vi "Main.vi"() -> ()   [LabVIEW 2016]
uses:
  <vilib>/Utility/error.llb/DialogType.ctl
  <vilib>/Utility/file.llb/Write Delimited Spreadsheet (string).vi
  <vilib>/Analysis/2dsp.llb/Rational Resample (single channel, DBL).vi
  <vilib>/measure/mamon.llb/Trigger Detection for 1 Channel.vi
  <vilib>/measure/NI_MAPro.lvlib
  <vilib>/Analysis/NI_AALPro.lvlib
panel:
  out "Waveform Graph":dbl[](graph)
  out "Y":dbl[](array[numeric])
  out "Software Version":string
  in  "Tab Control 2":enum32{"Calculated Values", "Other Values"}(tab)
  out "Contraction\nOnset (s)":dbl format="%_5g"
  out "Standing\nWeight":dbl format="%.1f"
  out "Peak Force":dbl format="%.1f"
  out "Mean Force":dbl format="%.1f"
  out "Min Force":dbl format="%.1f"
  out "TTPF":dbl format="%_5g"
  out "RFDPF":dbl format="%.1f"
  out "IMPPF":dbl format="%.1f"
  out "IMP250":dbl format="%_5g"
  out "IMP200":dbl format="%_5g"
  out "IMP150":dbl format="%_5g"
  out "IMP100":dbl format="%_5g"
  out "RFD250":dbl format="%.1f"
  out "RFD200":dbl format="%.1f"
  out "RFD150":dbl format="%.1f"
  out "RFD100":dbl format="%.1f"
  out "F250":dbl format="%.1f"
  out "F200":dbl format="%.1f"
  out "F150":dbl format="%.1f"
  out "F100":dbl format="%.1f"
  out "System Weight \nCursor Position":dbl
  out "Before Pull Cursor\nPosition":dbl
  out "After pull\nCursor Position":dbl
  out "SD of weighing period":dbl format="%#_4g"
  in  "stop 2":bool
  out "Index of min SD":dbl format="%#.2f"
  out "Minimum SD":dbl
  in  "Tab Control 3":T1(tab)
  out "Peak Deviation >50N\nfrom Average?":bool
  out "System Weight Segment":dynamicdata(graph)
  out "SW Segment Range":dbl
  out "Contraction Onset ID":dbl[](graph) caption="Section"
  out "Intra-Cursor Segment":dbl[](graph)
  in  "Tab Control":T2(tab)
  in  "Subject Body Mass (kg)":dbl
  in  "Subject Identifier (ID# or Last Name, First)":string
  in  "Trial Number":string
  in  "Trial Notes":string
  in  "Create Blank\nSave File":bool
  in  "Save Results":bool
  out "Target File for Saving Results":path
  in  "Choose New \nSave Target":bool
  out "Analysis File and File Path":path
  in  "Load File":bool
  in  "Sampling Rate\nof Force Signal":i32=100 min=100 max=2000 step=1 format="%#.0f"
  in  "Custom Onset Threshold\nValue in Newtons (SW+Threshold)":dbl min=0.0 max=500.0
  in  "# of Samples Averaged for system \nweight (Default is 1000).":i32=1000 caption="Samples" min=3 max=2000
  in  "Suppress \nData Prompt":bool
  in  "Contraction Onset ID Method":u16(ring) items=["5SD of Weighing", "20 N", "75 N", "Manual Identification", "Custom Threshold"]
  out "Force-time trace":dynamicdata(graph)
  # "Isometric Analyzer\nBy George Beckham, PhD"
  # "Main Github Repository: \nhttps://github.com/excellentsport/IsometricAnalyzer"
  # "This is beta version software, and may have bugs. \nPlease submit any that you find at: \nhttps://github.com/excellentsport/IsometricAnalyzer/issues"
  # "How to use: \nhttps://github.com/excellentsport/IsometricAnalyzer"
  # "All values displayed above are assumed to operate using Newtons as the unit of force. Hence, all boxes with force are\nin Newtons, all Rate of Force Development (RFD) are in Newtons per second (N/s), and Impulse (IMP) is in N•s.\n\nEach time specific value (e.g. F100) is calculated relative to the contraction onset (e.g. F100 is the force at 100ms after the contraction began)."
  # "Horizontal line is SW value"
  # "Green Cursor Designates the identified start of the push/pull\nRed Cursor Designates the identified end of the push/pull"
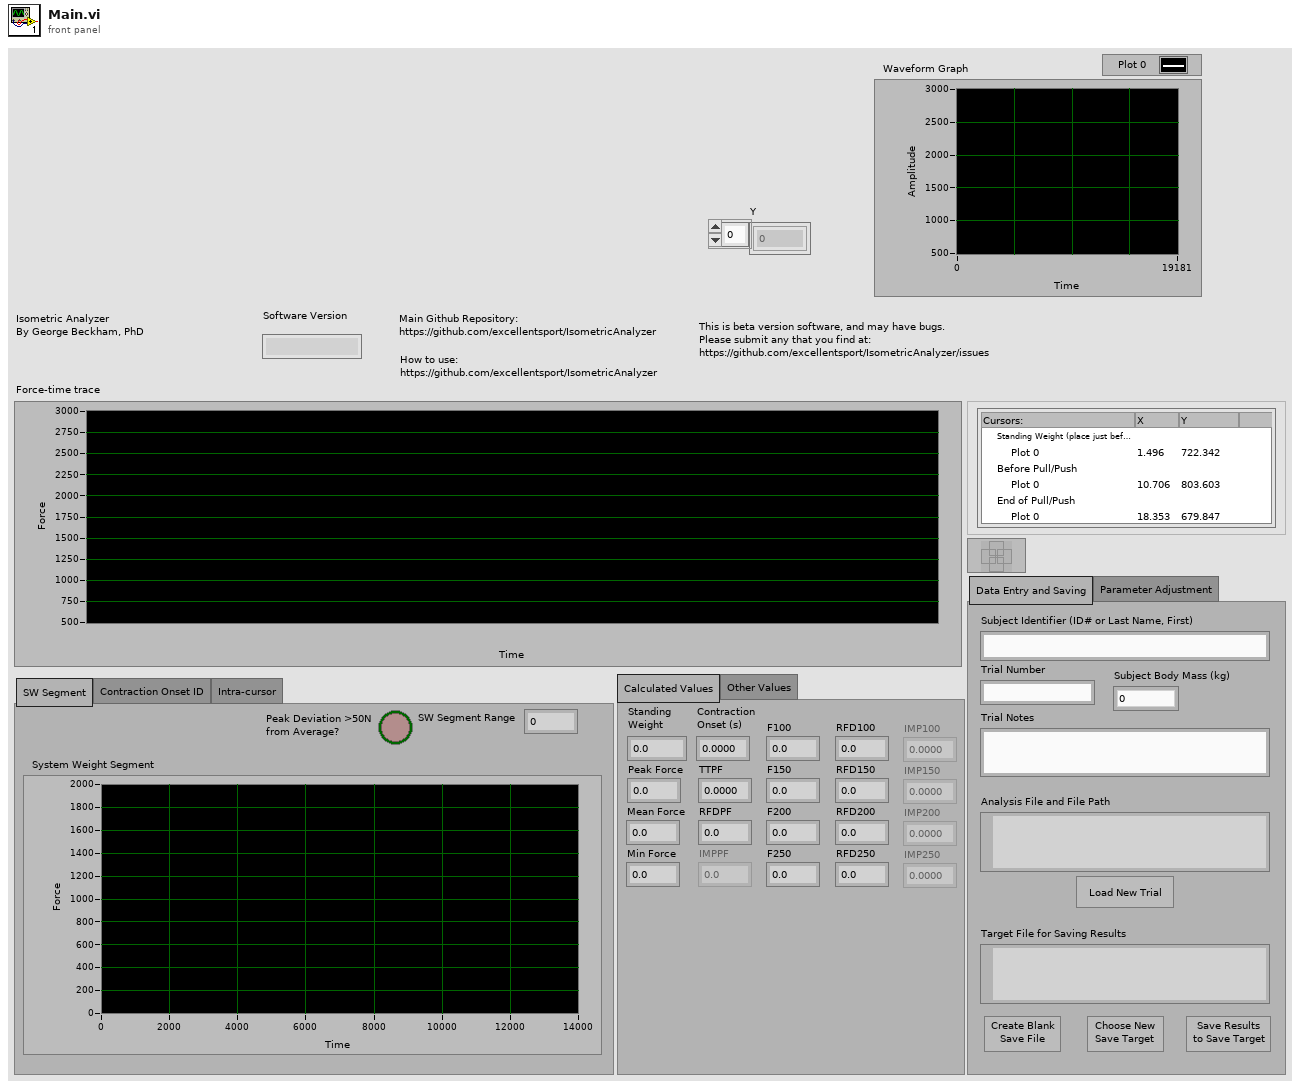
[diagram p1: front panel]
types:
  T1 = enum32{"SW Segment", "Contraction Onset ID", "Intra-cursor"}
  T2 = enum32{"Data Entry and Saving", "Parameter Adjustment"}
  T3 = typedef "DialogType.ctl" = u16
  T4 = cluster{i32, "Sampling Rate\nof Force Signal":i32}
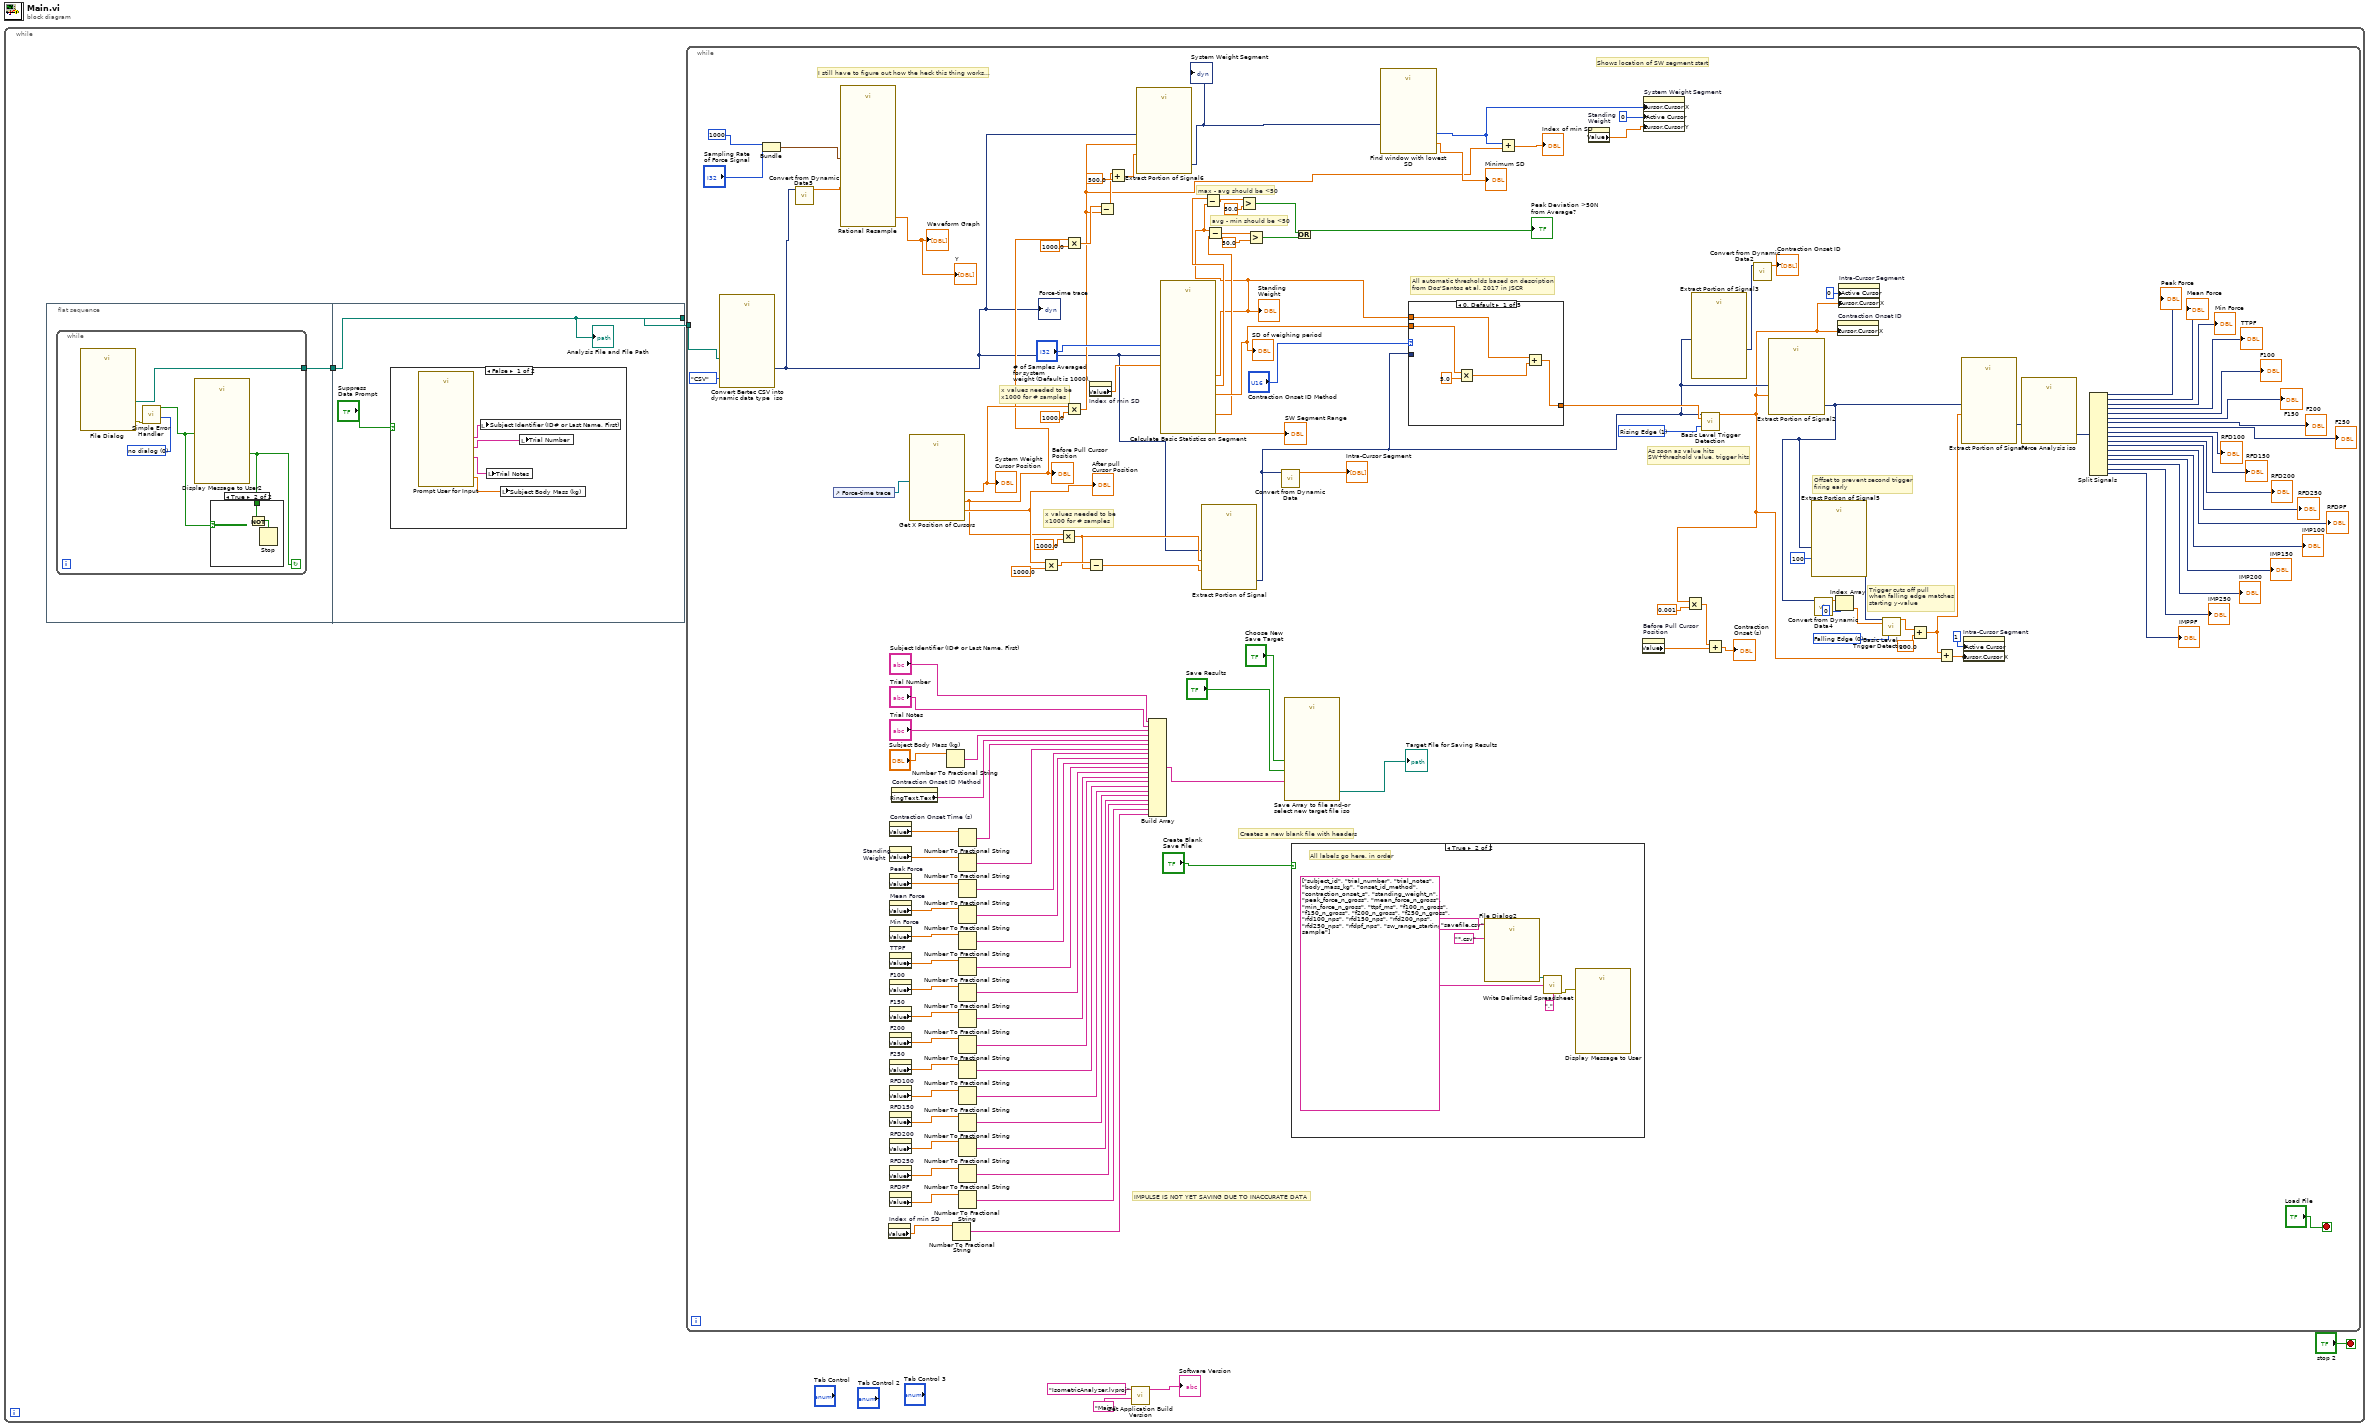
[diagram p0: block diagram]
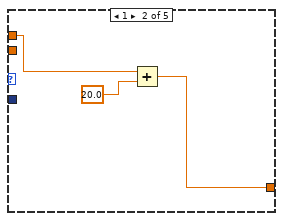
[diagram p4: hidden frame]
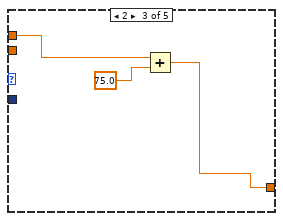
[diagram p5: hidden frame]
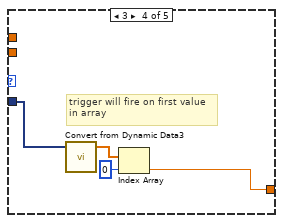
[diagram p6: hidden frame]
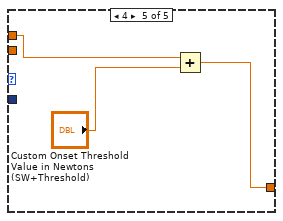
[diagram p7: hidden frame]
diagram:
  n1 = while {
    stop <- "stop 2" stop-if-true
    n2 = flat-sequence {
      tunnel: [w7] -> w1
      tunnel: [w15] -> w6
      tunnel: w1 -> [w15]
      frame #0 {
        n3 = while {
          tunnel: [w12] -> w7
          stop <- w9 continue-if-true
          w10 = T3 0 items=["no dialog", "OK message", "continue or stop message", "OK message + warnings", "continue/stop + warnings"] ("type of dialog (OK msg:1)")
          n4 = call "File Dialog"() -> ("selected path"=w12:path, "error out"=w11:errorcluster)  [unwired: 12 in, 2 out]
          n5 = call <vilib>:"Simple Error Handler.vi"("type of dialog (OK msg:1)"=w10, "error in (no error)"=w11) -> ("error?"=w8:bool)  [unwired: 3 in, 4 out]
          n6 = call "Display Message to User2"("Enable"=w8) -> ("OK"=w9:bool)  [unwired: 9 in, 1 out]
          n7 = case shown="True" w8 {
            tunnel: w9 -> [_ w13]
            frame False {
            }
            frame True {
              n8 = Not(x=w13) -> (.not. x?=w14:bool)
              n9 = Stop(stop? (T)=w14) -> ()
            }
          }
        }
      }
      frame #1 {
        n10 = case shown="False" "Suppress \nData Prompt" {
          frame False {
            n11 = call "Prompt User for Input"() -> ("Subject's body mass (kg)"=w17:dbl, "Trial Notes"=w19:string, "Trial Number"=w18:string, "Subject ID (e.g. 007) or Last Name, First Name"=w20:string)  [unwired: 14 in, 2 out]
            n12 = local write "Subject Identifier (ID# or Last Name, First)"(w20) -> ()
            n13 = local write "Trial Notes"(w19) -> ()
            n14 = local write "Subject Body Mass (kg)"(w17) -> ()
            n15 = local write "Trial Number"(w18) -> ()
          }
          frame True {
          }
        }
        "Analysis File and File Path" <- w15
      }
    }
    n16 = while {
      tunnel: w6 -> [w152]
      stop <- "Load File" stop-if-true
      w86 = u16 0 items=["Falling Edge", "Rising Edge"] ("trigger slope")
      w89 = u16 1 items=["Falling Edge", "Rising Edge"] ("trigger slope")
      # "I still have to figure out how the heck this thing works..."
      # "Shows location of SW segment start"
      # "Offset to prevent second trigger\nfiring early"
      # "avg - min should be <50"
      # "max - avg should be <50"
      # "All automatic thresholds based on description \nfrom Dos'Santos et al. 2017 in JSCR"
      # "Trigger cuts off pull\nwhen falling edge matches \nstarting y-value"
      # "As soon as value hits \nSW+threshold value, trigger hits"
      # "IMPULSE IS NOT YET SAVING DUE TO INACCURATE DATA"
      # "Creates a new blank file with headers"
      # "x values needed to be \nx1000 for # samples"
      # "x values needed to be \nx1000 for # samples"
      n17 = call "Convert Bertec CSV into dynamic data type  iso.vi"("selected path"=w152, "Input Datafile Separator"=enum32{"CSV", "TSV"}."CSV" ("Input Datafile Type")) -> ("Dynamic Data Type"=w26:dynamicdata)
      "Force-time trace" <- w26
      n18 = Bundle(1000, "Sampling Rate\nof Force Signal"="Sampling Rate\nof Force Signal") -> (w22:T4)  [unwired: 1 in]
      n19 = call "Convert from Dynamic Data5"("Dynamic Data Type"=w26) -> ("Array"=w25:dbl[])  [unwired: 3 in]
      n20 = control-ref of="Force-time trace"() -> (w150:refnum<vi>)
      n21 = call-poly <vilib>:"Rational Resample.vi"("resample factor"=w22, "X"=w25) -> ("Y"=→"Y" →"Waveform Graph":dbl[])  [unwired: 7 in, 2 out]
      n22 = property on="Index of min SD" class="DigNum (strict)"() -> ("Value"=w28:dbl)  [unwired: 2 in, 2 out]
      n23 = property on="Contraction Onset Time (s)" class="DigNum (strict)"() -> ("Value"=w61:dbl)  [unwired: 2 in, 2 out]
      n24 = property on="Standing\nWeight" class="DigNum (strict)"() -> ("Value"=w94:dbl)  [unwired: 2 in, 2 out]
      n25 = property on="Peak Force" class="DigNum (strict)"() -> ("Value"=w120:dbl)  [unwired: 2 in, 2 out]
      n26 = property on="Mean Force" class="DigNum (strict)"() -> ("Value"=w118:dbl)  [unwired: 2 in, 2 out]
      n27 = property on="Min Force" class="DigNum (strict)"() -> ("Value"=w117:dbl)  [unwired: 2 in, 2 out]
      n28 = property on="TTPF" class="DigNum (strict)"() -> ("Value"=w116:dbl)  [unwired: 2 in, 2 out]
      n29 = property on="F100" class="DigNum (strict)"() -> ("Value"=w115:dbl)  [unwired: 2 in, 2 out]
      n30 = property on="F150" class="DigNum (strict)"() -> ("Value"=w114:dbl)  [unwired: 2 in, 2 out]
      n31 = property on="F200" class="DigNum (strict)"() -> ("Value"=w113:dbl)  [unwired: 2 in, 2 out]
      n32 = property on="F250" class="DigNum (strict)"() -> ("Value"=w112:dbl)  [unwired: 2 in, 2 out]
      n33 = property on="RFD100" class="DigNum (strict)"() -> ("Value"=w111:dbl)  [unwired: 2 in, 2 out]
      n34 = property on="RFD150" class="DigNum (strict)"() -> ("Value"=w110:dbl)  [unwired: 2 in, 2 out]
      n35 = property on="RFD200" class="DigNum (strict)"() -> ("Value"=w109:dbl)  [unwired: 2 in, 2 out]
      n36 = property on="RFD250" class="DigNum (strict)"() -> ("Value"=w108:dbl)  [unwired: 2 in, 2 out]
      n37 = property on="RFDPF" class="DigNum (strict)"() -> ("Value"=w107:dbl)  [unwired: 2 in, 2 out]
      n38 = property on="Contraction Onset ID Method" class="Ring (strict)"() -> ("RingText.Text"=w52:string)  [unwired: 2 in, 2 out]
      n39 = call "Get X Position of Cursors.vi"("WaveformGraph in"=w150) -> ("Cursor 3 X Pos"=w91:dbl, "Cursor 2 X Pos"=w40:dbl, "Cursor 1 X Pos"=w92:dbl)  [unwired: 7 in]
      "After pull\nCursor Position" <- w91
      "Before Pull Cursor\nPosition" <- w40
      "System Weight \nCursor Position" <- w92
      n40 = Number To Fractional String(number="Subject Body Mass (kg)") -> (F-format string=w54:string)  [unwired: 3 in]
      n41 = Number To Fractional String(number=w28) -> (F-format string=w27:string)  [unwired: 3 in]
      n42 = Number To Fractional String(number=w61) -> (F-format string=w60:string)  [unwired: 3 in]
      n43 = Number To Fractional String(number=w94) -> (F-format string=w82:string)  [unwired: 3 in]
      n44 = Number To Fractional String(number=w120) -> (F-format string=w119:string)  [unwired: 3 in]
      n45 = Number To Fractional String(number=w118) -> (F-format string=w106:string)  [unwired: 3 in]
      n46 = Number To Fractional String(number=w117) -> (F-format string=w105:string)  [unwired: 3 in]
      n47 = Number To Fractional String(number=w116) -> (F-format string=w104:string)  [unwired: 3 in]
      n48 = Number To Fractional String(number=w115) -> (F-format string=w103:string)  [unwired: 3 in]
      n49 = Number To Fractional String(number=w114) -> (F-format string=w102:string)  [unwired: 3 in]
      n50 = Number To Fractional String(number=w113) -> (F-format string=w101:string)  [unwired: 3 in]
      n51 = Number To Fractional String(number=w112) -> (F-format string=w100:string)  [unwired: 3 in]
      n52 = Number To Fractional String(number=w111) -> (F-format string=w99:string)  [unwired: 3 in]
      n53 = Number To Fractional String(number=w110) -> (F-format string=w98:string)  [unwired: 3 in]
      n54 = Number To Fractional String(number=w109) -> (F-format string=w97:string)  [unwired: 3 in]
      n55 = Number To Fractional String(number=w108) -> (F-format string=w96:string)  [unwired: 3 in]
      n56 = Number To Fractional String(number=w107) -> (F-format string=w95:string)  [unwired: 3 in]
      n57 = Multiply(x=w91, y=1000.0) -> (x*y=w146:dbl)
      n58 = Multiply(x=w40, y=1000.0) -> (x*y=w42:dbl)
      n59 = Multiply(x=w40, y=1000.0) -> (x*y=w38:dbl)
      n60 = Multiply(x=w92, y=1000.0) -> (x*y=w36:dbl)
      n61 = Subtract(x=w146, y=w42) -> (x-y=w145:dbl)
      n62 = property on="Index of min SD" class="DigNum (strict)"() -> ("Value"=w34:dbl)  [unwired: 2 in, 2 out]
      n63 = Subtract(x=w38, y=w36) -> (x-y=w41:dbl)
      n64 = Add(x=w41, y=500.0) -> (x+y=w44:dbl)
      n65 = call "Extract Portion of Signal6"("Samples"=w44, "Begin Sample"=w36, "Signals"=w26) -> ("Section"=w33:dynamicdata)  [unwired: 7 in, 1 out]
      "System Weight Segment" <- w33
      n66 = Build Array("Subject Identifier (ID# or Last Name, First)", "Trial Number", "Trial Notes", w54, w52, w60, w82, w119, w106, w105, w104, w103, w102, w101, w100, w99, w98, w97, w96, w95, w27) -> (w123:string[])
      n67 = call "Calculate Basic Statistics on Segment.vi"("# of Samples Averaged\nfor standing weight\n(1000 is default)"="# of Samples Averaged for system \nweight (Default is 1000).", "Start of Sample"=w34, "Dynamic Data Type"=w26) -> ("Minimum"=w70:dbl, "Maximum"=w69:dbl, "Standard Deviation"=w83:dbl, "Arithmetic Mean"=w29:dbl, "Range"=→"SW Segment Range":dbl)  [unwired: 3 in, 1 out]
      "Standing\nWeight" <- w29
      "SD of weighing period" <- w83
      n68 = call "Extract Portion of Signal"("Samples"=w145, "Begin Sample"=w42, "Signals"=w26) -> ("Section"=w79:dynamicdata)  [unwired: 7 in, 1 out]
      n69 = Subtract(x=w69, y=w29) -> (x-y=w71:dbl)
      n70 = Subtract(x=w29, y=w70) -> (x-y=w66:dbl)
      n71 = Greater?(x=w71, y=50.0) -> (0:w73:bool)
      n72 = Greater?(x=w66, y=50.0) -> (0:w68:bool)
      n73 = call "Convert from Dynamic Data"("Dynamic Data Type"=w79) -> ("Array"=→"Intra-Cursor Segment":dbl[])  [unwired: 3 in]
      n74 = call "Save Array to file and-or select new target file iso.vi"("Choose New \nSave Target"="Choose New \nSave Target", "Save Results"="Save Results", "Values to Save"=w123) -> ("selected path"=→"Target File for Saving Results":path)  [unwired: 8 in]
      n75 = case shown="True" "Create Blank\nSave File" {
        frame False {
        }
        frame True {
          # "All labels go here, in order"
          n76 = call "File Dialog2"("default name"="savefile.csv", "pattern (all files)"="*.csv") -> ("selected path"=w174:path)  [unwired: 10 in, 3 out]
          n77 = call-poly <vilib>:"Write Delimited Spreadsheet.vi"("file path (dialog if empty)"=w174, "1D data"=string[] ["subject_id", "trial_number", "trial_notes", "body_mass_kg", "onset_id_method", "contraction_onset_s", "standing_weight_n", "peak_force_n_gross", "mean_force_n_gross", "min_force_n_gross", "ttpf_ms", "f100_n_gross", "f150_n_gross", "f200_n_gross", "f250_n_gross", "rfd100_nps", "rfd150_nps", "rfd200_nps", "rfd250_nps", "rfdpf_nps", "sw_range_starting_sample"], "delimiter (\\t)"="," ("delimiter (\\t)")) -> ("error out"=w176:errorcluster)  [unwired: 11 in, 1 out]
          n78 = call "Display Message to User"("error in (no error)"=w176) -> ()  [unwired: 9 in, 2 out]
        }
      }
      n79 = Or(x=w73, y=w68) -> (x .or. y?=→"Peak Deviation >50N\nfrom Average?":bool)
      n80 = call "Find window with lowest SD.vi"("Input Data"=w33) -> ("Index of min SD"=w32:i32, "Minimum SD"=→"Minimum SD":dbl)  [unwired: 9 in]
      n81 = case shown="0, Default" "Contraction Onset ID Method" {
        tunnel: w79 -> [_ _ _ w166 _]
        tunnel: [w158 w159 w162 w165 w169] -> w84
        tunnel: w29 -> [w157 w161 w163 _ w171]
        tunnel: w83 -> [w154 _ _ _ _]
        frame 0, Default {
          n82 = Multiply(x=w154, y=5.0) -> (x*y=w156:dbl)
          n83 = Add(x=w157, y=w156) -> (x+y=w158:dbl)
        }
        frame 1 {
          n84 = Add(x=w161, y=20.0) -> (x+y=w159:dbl)
        }
        frame 2 {
          n85 = Add(x=w163, y=75.0) -> (x+y=w162:dbl)
        }
        frame 3 {
          # "trigger will fire on first value\nin array"
          n86 = call "Convert from Dynamic Data3"("Dynamic Data Type"=w166) -> ("Array"=w167:dbl[])  [unwired: 3 in]
          n87 = Index Array(array=w167, index=0) -> (element=w165:dbl)
        }
        frame 4 {
          n88 = Add(x=w171, y="Custom Onset Threshold\nValue in Newtons (SW+Threshold)") -> (x+y=w169:dbl)
        }
      }
      n89 = Add(x=w32, y=w36) -> (x+y=→"Index of min SD":dbl)
      n90 = property on="Standing\nWeight" class="DigNum (strict)"() -> ("Value"=w31:dbl)  [unwired: 2 in, 2 out]
      n91 = property on="Before Pull Cursor\nPosition" class="DigNum (strict)"() -> ("Value"=w62:dbl)  [unwired: 2 in, 2 out]
      n92 = property on="System Weight Segment" class="WFGraph (strict)"("Cursor.Cursor X"=w32, "Active Cursor"=u32 0, "Cursor.Cursor Y"=w31) -> ()  [unwired: 2 in, 2 out]
      n93 = call "Extract Portion of Signal3"("Signals"=w79) -> ("Section"=w88:dynamicdata)  [unwired: 9 in, 1 out]
      n94 = call-poly <vilib>:"Basic Level Trigger Detection.vi"("signal in"=w79, "level"=w84, "trigger slope"=w89) -> ("trigger location"=w51:dbl)  [unwired: 10 in, 2 out]
      n95 = Multiply(x=w51, y=0.001) -> (x*y=w63:dbl)
      n96 = Add(x=w63, y=w62) -> (x+y=→"Contraction\nOnset (s)":dbl)
      n97 = call "Convert from Dynamic Data2"("Dynamic Data Type"=w88) -> ("Array"=→"Contraction Onset ID":dbl[])  [unwired: 3 in]
      n98 = call "Extract Portion of Signal2"("Begin Sample"=w51, "Signals"=w79) -> ("Section"=w50:dynamicdata)  [unwired: 8 in, 1 out]
      n99 = call "Extract Portion of Signal5"("Begin Sample"=100, "Signals"=w50) -> ("Section"=w48:dynamicdata)  [unwired: 8 in, 1 out]
      n100 = call "Convert from Dynamic Data4"("Dynamic Data Type"=w50) -> ("Array"=w78:dbl[])  [unwired: 3 in]
      n101 = Index Array(array=w78, index=0) -> (element=w76:dbl)
      n102 = property on="Contraction Onset ID" class="WFGraph (strict)"("Cursor.Cursor X"=w51) -> ()  [unwired: 2 in, 2 out]
      n103 = property on="Intra-Cursor Segment" class="WFGraph (strict)"("Active Cursor"=u32 0, "Cursor.Cursor X"=w51) -> ()  [unwired: 2 in, 2 out]
      n104 = call-poly <vilib>:"Basic Level Trigger Detection.vi"("signal in"=w48, "level"=w76, "trigger slope"=w86) -> ("trigger location"=w46:dbl)  [unwired: 10 in, 2 out]
      n105 = Add(x=w46, y=100.0) -> (x+y=w47:dbl)
      n106 = Add(x=w47, y=w51) -> (x+y=w75:dbl)
      n107 = call "Extract Portion of Signal4"("Samples"=w47, "Signals"=w50) -> ("Section"=w85:dynamicdata)  [unwired: 8 in, 1 out]
      n108 = property on="Intra-Cursor Segment" class="WFGraph (strict)"("Active Cursor"=u32 1, "Cursor.Cursor X"=w75) -> ()  [unwired: 2 in, 2 out]
      n109 = call "Force Analysis iso.vi"("Dynamic Data Type 2"=w85) -> ("Dynamic Data Type"=w144:dynamicdata)
      n110 = Split Signals(w144) -> (→"Peak Force":dynamicdata, →"Mean Force":dynamicdata, →"Min Force":dynamicdata, →"TTPF":dynamicdata, →"F100":dynamicdata, →"F150":dynamicdata, →"F200":dynamicdata, →"F250":dynamicdata, →"RFD100":dynamicdata, →"RFD150":dynamicdata, →"RFD200":dynamicdata, →"RFD250":dynamicdata, →"RFDPF":dynamicdata, →"IMP100":dynamicdata, →"IMP150":dynamicdata, →"IMP200":dynamicdata, →"IMP250":dynamicdata, →"IMPPF":dynamicdata)  [unwired: 18 in]
    }
    n111 = call "Get Application Build Version.vi"("Build Specification Name"="Main", "Project Filename"="IsometricAnalyzer.lvproj") -> ("Version String"=→"Software Version":string)  [unwired: 7 in, 2 out]
  }
